vi "Create and Read PWM Output.vi"(8 "error in":errorcluster, 10 "channel settings in":T1[](array[typedef]), 11 "module test in":refnum<class "Module Test.lvclass">) -> (0 "error out":errorcluster, 2 "channel settings out":T1[](array[typedef]), 3 "module test out":refnum<class "Module Test.lvclass">)   [LabVIEW 2020, in "Module Test.lvclass"]
uses:
  Module Test.lvclass
  Scripting/Modules/Mode Classes/Controls/pwm channel settings.ctl
  Scripting/Modules/Channel Classes/PWM Output Channel/Frequency.ctl
  Scripting/Modules/Channel Classes/PWM Output Channel/PWM Output Channel.lvclass
  Scripting/Scan Engine Scripting.lvlib
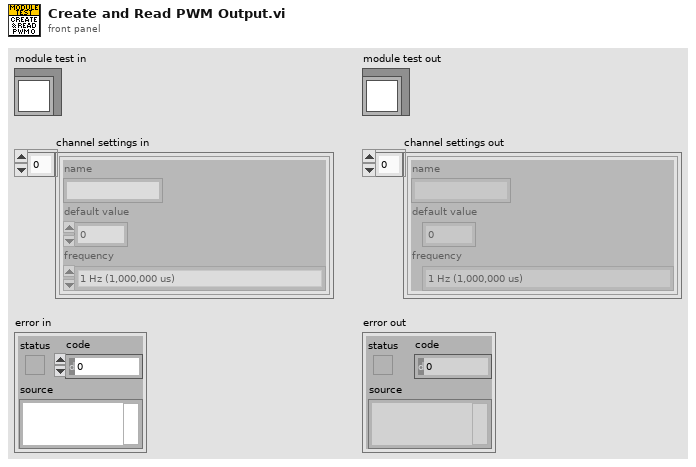
[diagram p1: front panel]
types:
  T1 = typedef "Scan Engine Scripting.lvlib/pwm channel settings.ctl" = cluster{"name":string, "default value":dbl, "frequency":T2}
  T2 = typedef "Scan Engine Scripting.lvlib/PWM Output Channel.lvclass/Frequency.ctl" = enum16{"1 Hz (1,000,000 us)", "50 Hz (20,000 us)", "250 Hz (4,000 us)", "500 Hz (2,000 us)", "1 kHz (1,000 us)", "5 kHz (200 us)", "10 kHz (100 us)", "20 kHz (50 us)"}
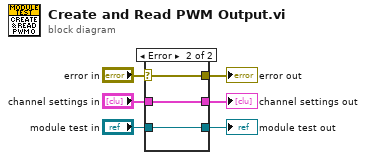
[diagram p0: block diagram]
diagram:
  n1 = case shown="Error" "error in" {
    selector: "error in" -> [w8 w12]
    tunnel: [w8 w12] -> w5
    tunnel: [w9 w11] -> w3
    tunnel: "module test in" -> [w9 w11]
    tunnel: "channel settings in" -> [w7 w10]
    tunnel: [w7 w10] -> w1
    frame No Error {
    }
    frame Error {
    }
  }
  "error out" <- w5
  "module test out" <- w3
  "channel settings out" <- w1
